vi "HighLvCtrl_Init.vi"(8 "error in (no error)":errorcluster, 11 "CAlexVersion":T1=enum."Mobile") -> (0 "error out":errorcluster, 3 "HighLvClasses":T3={"CAlexVersion"=enum."Mobile", "CAlex2 out"=refnum, "ForceField"=refnum})   [LabVIEW 2016]
uses:
  TypeDef/HighLvControl Cluster.ctl
  Classes/CAlex2/CAlex2.lvclass
  Classes/ForceField/ForceField.lvclass
  Classes/CAlex2/TypeDef/CAlexVersion.ctl
  Classes/CAlex2/TypeDef/LowerBodyDim.ctl
panel:
  in  "dt":dbl=0.005 format="%#_13g"
  in  "LegProperties":T2={"BodyDim"={"ThighLt (m)"=0.4, "ShankLt (m)"=0.41, "HipWd (m)"=0.32}, "BodyWt"={"Thigh (kg)"=0.0, "Shank (kg)"=0.0}, "Cuff Loc"={"HipCuffWd (m)"=0.4, "HipCuffHt (m)"=0.1, "HipFwdShift (m)"=0.0, "ThighToKnee (m)"=0.25, "ThighCuffDist (m)"=0.0254, "ShankToKnee (m)"=0.15}}
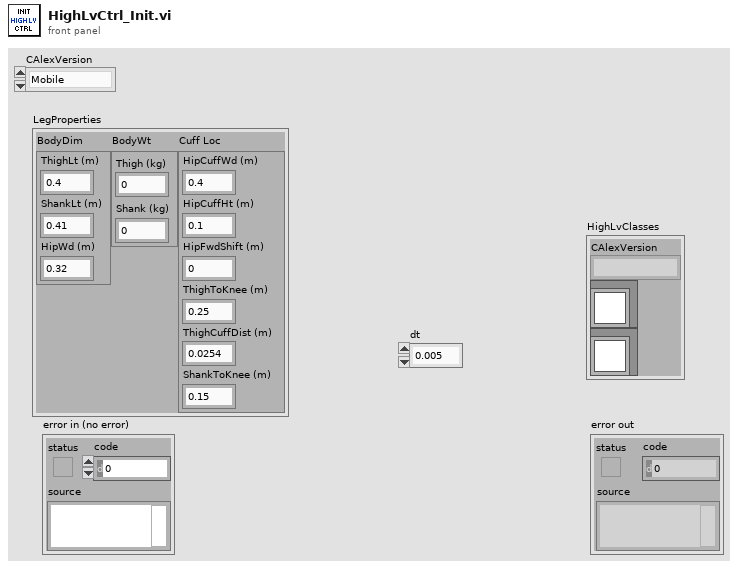
[diagram p1: front panel]
types:
  T1 = typedef "CAlex2.lvclass/CAlexVersion.ctl" = enum16{"Bilateral_Squat", "Treadmill", "Mobile"}
  T2 = typedef "CAlex2.lvclass/LowerBodyDim.ctl" = cluster{"BodyDim":cluster{"ThighLt (m)":dbl, "ShankLt (m)":dbl, "HipWd (m)":dbl}, "BodyWt":cluster{"Thigh (kg)":dbl, "Shank (kg)":dbl}, "Cuff Loc":cluster{"HipCuffWd (m)":dbl, "HipCuffHt (m)":dbl, "HipFwdShift (m)":dbl, "ThighToKnee (m)":dbl, "ThighCuffDist (m)":dbl, "ShankToKnee (m)":dbl}}
  T3 = typedef "HighLvControl Cluster.ctl" = cluster{"CAlexVersion":T1, "CAlex2 out":refnum<class "CAlex2.lvclass">, "ForceField":refnum<class "ForceField.lvclass">}
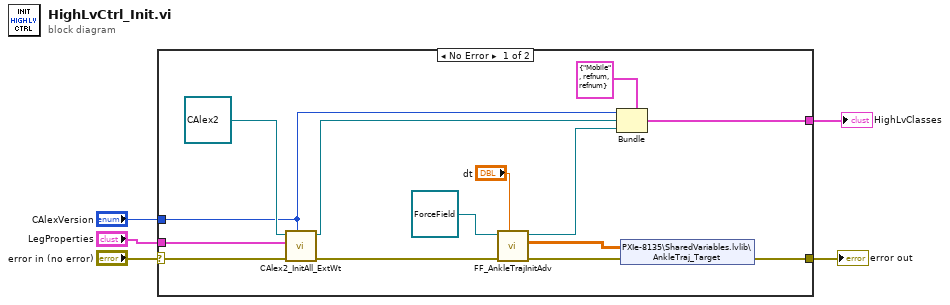
[diagram p0: block diagram]
diagram:
  n1 = case shown="No Error" "error in (no error)" {
    selector: "error in (no error)" -> [w11 w20]
    tunnel: [w19 _] -> w5
    tunnel: "LegProperties" -> [w18 _]
    tunnel: [w12 w20] -> w3
    tunnel: "CAlexVersion" -> [w7 _]
    frame No Error {
      n2 = call "CAlex2_InitAll_ExtWt.vi"("CAlexVersion"=w7, "error in (no error)"=w11, "LegProperties"=w18, "CAlex2 in"=refnum<class "CAlex2.lvclass"> refnum ("CAREX_NYU")) -> ("error out"=w16:errorcluster, "CAlex2 out"=w9:refnum<class "CAlex2.lvclass">)  [unwired: 6 in]
      n3 = call "FF_AnkleTrajInitAdv.vi"("dt (0.01)"="dt", "error in (no error)"=w16, "Force Field Controller in"=refnum<class "ForceField.lvclass"> refnum ("ForceField")) -> ("error out"=w13:errorcluster, "AnkleTraj dup"=w14:dbl[][], "Force Field Controller out"=w15:refnum<class "ForceField.lvclass">)  [unwired: 6 in]
      n4 = Bundle(cluster=T3 {"CAlexVersion"=enum."Mobile", "CAlex2 out"=refnum, "ForceField"=refnum} ("HighLvClasses"), "CAlexVersion"=w7, "CAlex2 out"=w9, "ForceField"=w15) -> (w19:T3)
      n5 = shared-variable "PXIe-8135\\SharedVariables.lvlib\\AnkleTraj_Target"(w14, error in=w13) -> (error out=w12:errorcluster)
    }
    frame Error {
    }
  }
  "error out" <- w3
  "HighLvClasses" <- w5
